vi "Get PDO Mappable Entries.vi"(8 "error in":errorcluster, 11 "Electronic Datasheet in":refnum<class "Electronic Datasheet.lvclass">) -> (0 "error out":errorcluster, 2 "PDO Mappable Entries":refnum<class "OD Entry.lvclass">[](array[class]), 3 "Electronic Datasheet out":refnum<class "Electronic Datasheet.lvclass">)   [LabVIEW 2020, in "Electronic Datasheet.lvlib" / "Electronic Datasheet.lvclass"]
uses:
  Electronic Datasheet.lvclass
  Electronic Datasheet.lvclass/Electronic Datasheet.ctl
  Core/OD Sub-Entry/OD Sub-Entry.lvclass
  Core/OD Entry/OD Entry.lvclass
  Core/Sorted Object Dictionary/Sorted Object Dictionary.lvclass
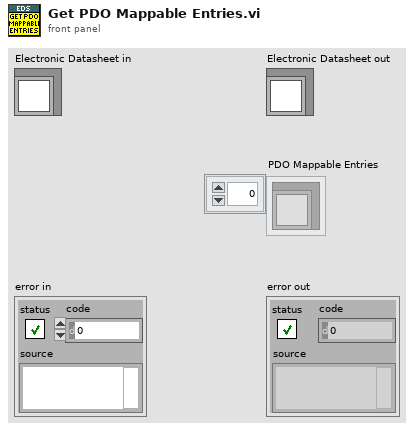
[diagram p1: front panel]
types:
  T1 = typedef "Electronic Datasheet.lvlib/Electronic Datasheet.lvclass/ObjectAttributes.ctl" = cluster{"EDS File Path":path, "Object Dict":refnum<class "Dictionary.lvclass">, "Sorted Object Dict":refnum<class "Sorted Object Dictionary.lvclass">, "Device Info":refnum<class "Device Info.lvclass">, "File Info":refnum<class "File Info.lvclass">}
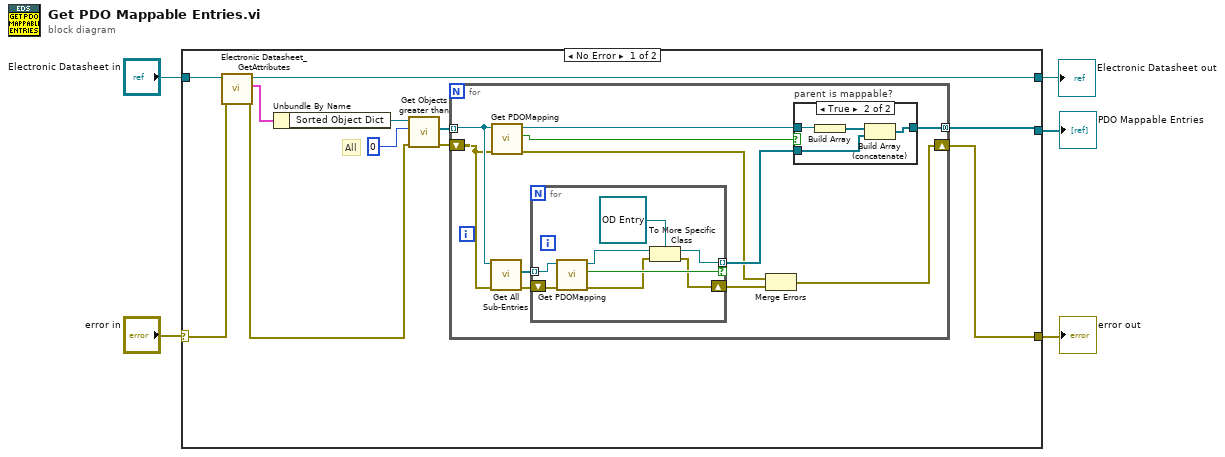
[diagram p0: block diagram]
diagram:
  n1 = case shown="No Error" "error in" {
    selector: "error in" -> [w16 w42]
    tunnel: [w7 w42] -> w4
    tunnel: [w14 w41] -> w2
    tunnel: "Electronic Datasheet in" -> [w15 w41]
    tunnel: [w12 _] -> w1
    frame No Error {
      # "All"
      n2 = call "Electronic Datasheet_GetAttributes.vi"("Error In"=w16, "reference in"=w15) -> ("Error Out"=w13:errorcluster, "Data"=w8:T1, "reference out"=w14:refnum<class "Electronic Datasheet.lvclass">)  [unwired: 6 in, 1 out]
      n3 = Unbundle By Name(w8) -> ("Sorted Object Dict"=w11:refnum<class "Sorted Object Dictionary.lvclass">)
      n4 = call "Get Objects greater than.vi"("error in"=w13, "Lower Bound"=u16 0, "Sorted Object Dictionary in"=w11) -> ("error out"=w9:errorcluster, "Entries"=w10:refnum<class "OD Entry.lvclass">[])  [unwired: 6 in, 1 out]
      n5 = for {
        tunnel: w10 -> [w26] mode=indexing
        tunnel: [w20] -> w12 mode=concatenating
        shift-right: [w17] -> w7
        shift-left: w9 -> [w25]
        n6 = call "Get All Sub-Entries.vi"("Error In"=w25, "reference in"=w26) -> ("Error Out"=w24:errorcluster, "Sub-Entries"=w23:refnum<class "OD Sub-Entry.lvclass">[])  [unwired: 6 in, 2 out]
        n7 = call "Get PDOMapping.vi"("Error In"=w25, "reference in"=w26) -> ("Error Out"=w19:errorcluster, "PDO Mapping?"=w27:bool, "reference out"=w22:refnum<class "OD Entry.lvclass">)  [unwired: 7 in]
        n8 = for {
          tunnel: w23 -> [w39] mode=indexing
          tunnel: [w36] -> w21 mode=indexing if=w37
          shift-right: [w33] -> w18
          shift-left: w24 -> [w40]
          n9 = call "Get PDOMapping.vi"("Error In"=w40, "reference in"=w39) -> ("Error Out"=w34:errorcluster, "PDO Mapping?"=w37:bool, "reference out"=w38:refnum<class "OD Sub-Entry.lvclass">)  [unwired: 7 in]
          n10 = To More Specific Class(target class=refnum<class "OD Entry.lvclass"> refnum ("Electronic Datasheet.lvlib:OD Entry"), reference=w38, error in=w34) -> (specific class reference=w36:refnum<class "OD Entry.lvclass">, error out=w33:errorcluster)
        }
        n11 = Merge Errors(w19, w18) -> (w17:errorcluster)
        n12 = case "parent is mappable?" shown="True" w27 {
          tunnel: w22 -> [_ w32]
          tunnel: w21 -> [w28 w30]
          tunnel: [w28 w29] -> w20
          frame False {
          }
          frame True {
            n13 = Build Array(w32) -> (w31:refnum<class "OD Entry.lvclass">[])
            n14 = Build Array (concatenate)(w31, w30) -> (w29:refnum<class "OD Entry.lvclass">[])
          }
        }
      }
    }
    frame Error {
    }
  }
  "error out" <- w4
  "Electronic Datasheet out" <- w2
  "PDO Mappable Entries" <- w1
